vi "Kikusui PLZ-Initialize.vi"(8 "error in":errorcluster, 10 "Reset":bool, 11 "Kikusui PLZ Setting In":T1={"VISA Resource Name"="", "Baud Rate"=19200, "Stop Bits"=20, "Wait For Read(ms)"=0} {"Stop Bits" items=["1.0"=10, "2.0"=20]; "Baud Rate" items=["2400"=2400, "4800"=4800, "9600"=9600, "19200"=19200]}) -> (0 "error out":errorcluster, 3 "Kikusui PLZ Setting Out":T1={"VISA Resource Name"="", "Baud Rate"=19200, "Stop Bits"=20, "Wait For Read(ms)"=0} {"Stop Bits" items=["1.0"=10, "2.0"=20]; "Baud Rate" items=["2400"=2400, "4800"=4800, "9600"=9600, "19200"=19200]})   [LabVIEW 2018]
doc: "Establishes communication with the instrument and optionally performs an instrument identification query and/or an instrument reset. It also places the instrument in a default state needed for other instrument driver operations. Therefore, call this VI before calling other instrument driver VIs for this instrument. Generally, you need to call the Initialize VI only once at the beginning of an application."
uses:
  Data Def/Kikusui PLZ-Setting.ctl
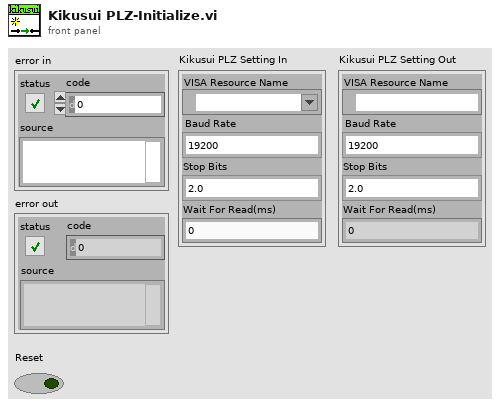
[diagram p1: front panel]
types:
  T1 = typedef "Kikusui PLZ-Setting.ctl" = cluster{"VISA Resource Name":refnum<visa-resource-name>, "Baud Rate":u32, "Stop Bits":u16, "Wait For Read(ms)":u32}
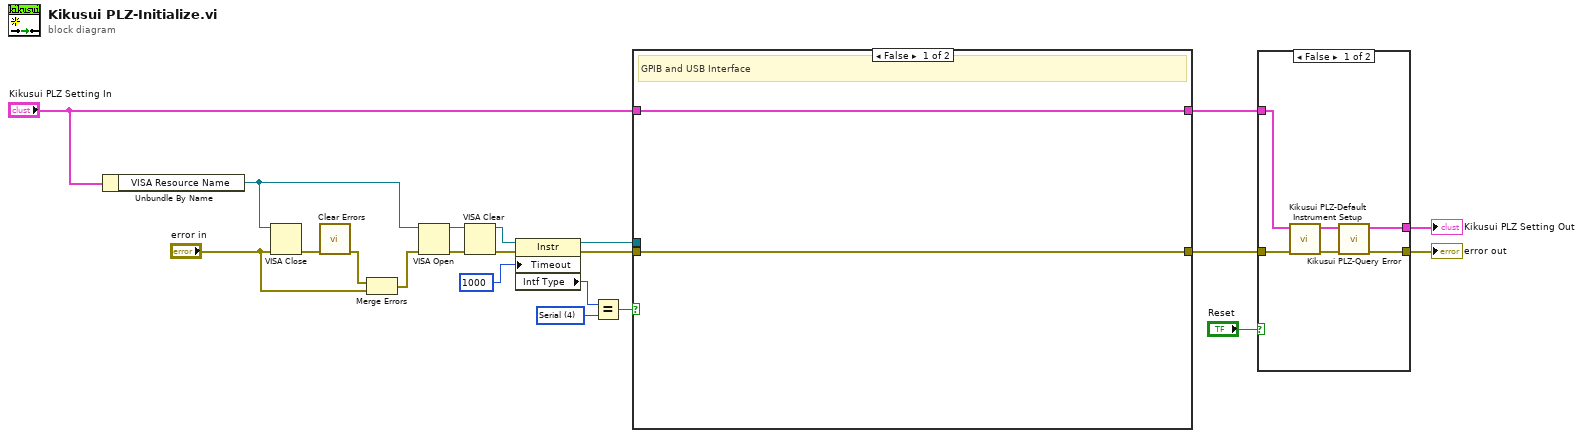
[diagram p0: block diagram]
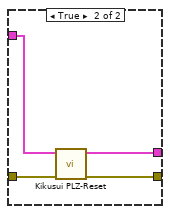
[diagram p2: hidden frame]
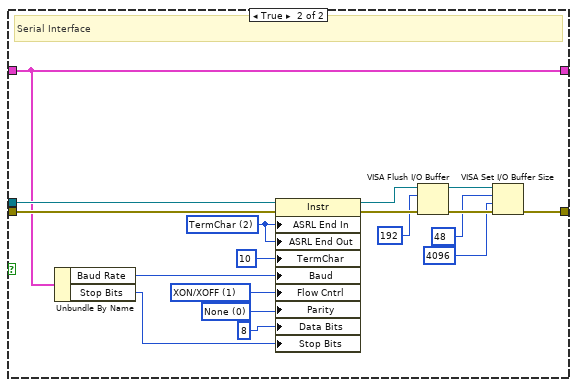
[diagram p3: hidden frame]
diagram:
  w12 = u16 4 items=["GPIB"=1, "VXI"=2, "GPIB-VXI"=3, "Serial"=4, "PXI"=5, "TCPIP"=6, "USB"=7] ("Interface Information:Interface Type")
  n1 = Unbundle By Name("Kikusui PLZ Setting In") -> ("VISA Resource Name"=w20:refnum<visa-resource-name>)
  n2 = VISA Close(VISA resource name=w20, error in (no error)="error in") -> (error out=w21:errorcluster)
  n3 = call <vilib>:"Clear Errors.vi"("error in (no error)"=w21) -> ("error out"=w6:errorcluster)  [unwired: 5 in, 1 out]
  n4 = Merge Errors(w6, "error in") -> (w4:errorcluster)
  n5 = VISA Open(error in (no error)=w4, VISA resource name=w20) -> (VISA resource name=w18:refnum<visa-resource-name>, error out=w19:errorcluster)  [unwired: 3 in]
  n6 = VISA Clear(VISA resource name=w18, error in (no error)=w19) -> (VISA resource name out=w16:refnum<visa-resource-name>, error out=w17:errorcluster)
  n7 = property class="Instr"(reference=w16, error in=w17, "Timeout"=u32 1000 ("General Settings:Timeout Value")) -> (reference out=w14:refnum<visa-resource-name>, error out=w15:errorcluster, "Intf Type"=w11:u16)
  n8 = Equal?(x=w11, y=w12) -> (x = y?=w10:bool)
  n9 = case shown="False" w10 {
    tunnel: w15 -> [w23 w34]
    tunnel: w14 -> [_ w33]
    tunnel: "Kikusui PLZ Setting In" -> [w22 w24]
    tunnel: [w23 w25] -> w8
    tunnel: [w22 w24] -> w2
    frame False {
      # "GPIB and USB Interface"
    }
    frame True {
      w28 = u16 0 items=["None", "Odd", "Even", "Mark", "Space"] ("Serial Settings:Parity")
      w29 = u16 1 items=["None", "XON/XOFF", "RTS/CTS", "XON/XOFF & RTS/CTS", "DTR/DSR", "XON/XOFF & DTR/DSR"] ("Serial Settings:Flow Control")
      w32 = u16 2 items=["None", "Last Bit", "TermChar"] ("Serial Settings:End Mode for Reads")
      # "Serial Interface"
      n10 = Unbundle By Name(w24) -> ("Baud Rate"=w30:u32, "Stop Bits"=w26:u16)
      n11 = property class="Instr"(reference=w33, error in=w34, "ASRL End In"=w32, "ASRL End Out"=w32, "TermChar"=u8 10 ("Message Based Settings:Termination Character"), "Baud"=w30, "Flow Cntrl"=w29, "Parity"=w28, "Data Bits"=u16 8 ("Serial Settings:Data Bits"), "Stop Bits"=w26) -> (reference out=w41:refnum<visa-resource-name>, error out=w40:errorcluster)
      n12 = VISA Flush I/O Buffer(VISA resource name=w41, mask (16)=u16 192, error in (no error)=w40) -> (VISA resource name out=w38:refnum<visa-resource-name>, error out=w39:errorcluster)
      n13 = VISA Set I/O Buffer Size(VISA resource name=w38, mask (16)=u16 48, size (4096)=u32 4096 ("size (0)"), error in (no error)=w39) -> (error out=w25:errorcluster)  [unwired: 1 out]
    }
  }
  n14 = case shown="False" "Reset" {
    tunnel: w8 -> [w47 w51]
    tunnel: [w44 w50] -> w7
    tunnel: [w43 w48] -> w1
    tunnel: w2 -> [w42 w49]
    frame False {
      n15 = call "Kikusui PLZ-Default Instrument Setup.vi"("error in"=w47, "Kikusui PLZ Setting In"=w42) -> ("error out"=w46:errorcluster, "Kikusui PLZ Setting Out"=w45:T1)  [unwired: 8 in]
      n16 = call "Kikusui PLZ-Query Error.vi"("error in"=w46, "Kikusui PLZ Setting In"=w45) -> ("error out"=w44:errorcluster, "Kikusui PLZ Setting Out"=w43:T1)  [unwired: 8 in]
    }
    frame True {
      n17 = call "Kikusui PLZ-Reset.vi"("error in"=w51, "Kikusui PLZ Setting In"=w49) -> ("error out"=w50:errorcluster, "Kikusui PLZ Setting Out"=w48:T1)  [unwired: 8 in]
    }
  }
  "error out" <- w7
  "Kikusui PLZ Setting Out" <- w1
